vi "CoordToMeters.vi"(10 "Ref Point":cluster{"Lat":dbl, "Long":dbl} {"Long" format="%#.22g"; "Lat" format="%#.22g"}, 11 "GPS position":cluster{"Lat":dbl, "Long":dbl} {"Long" format="%#.22g"; "Lat" format="%#.22g"}) -> (2 "X":dbl format="%#.14g", 3 "Y":dbl format="%#.14g")   [LabVIEW 2016]
uses:
  <vilib>/imath/engines/lvmath2/RunTimeEngine/NodeEndStatement/NIMS_NodeEndStatement_Output.vi
  <instcachedir>/0/NIMS_NodeEndStatement_Output_53EC0D466D134D7ABD903AC30B43404B.lvgen/NIMS_NodeEndStatement_Output_53EC0D466D134D7ABD903AC30B43404B_001.vi
  <vilib>/imath/engines/lvmath2/RunTimeEngine/ErrorHandling/NIMS_Finalize Error.vi
panel:
  out "Distance to the reference point":dbl format="%#.22g"
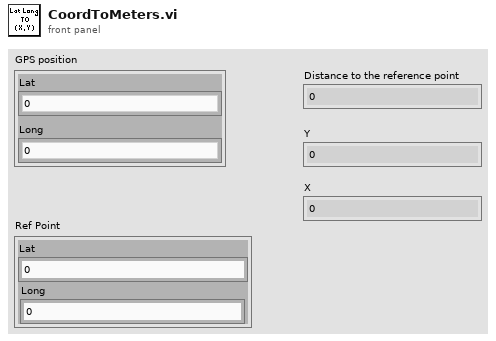
[diagram p1: front panel]
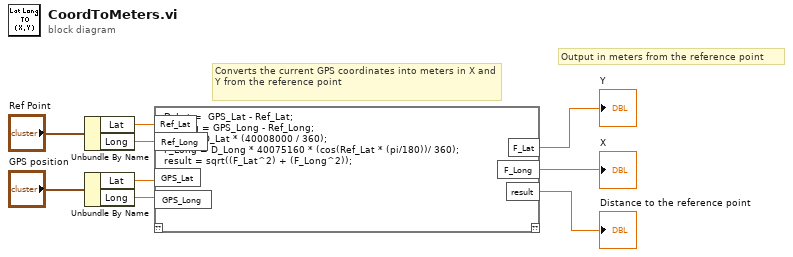
[diagram p0: block diagram]
diagram:
  # "Output in meters from the reference point"
  # "Converts the current GPS coordinates into meters in X and Y from the reference point"
  n1 = Unbundle By Name("Ref Point") -> ("Lat"=w6:dbl, "Long"=w5:dbl)
  n2 = Unbundle By Name("GPS position") -> ("Lat"=w2:dbl, "Long"=w1:dbl)
  n3 = mathscript code="D_Lat =  GPS_Lat - Ref_Lat;\nD_Long = GPS_Long - Ref_Long;\nF_Lat = D_Lat * (40008000 / 360);\nF_Long = D_Long * 40075160 * (cos(Ref_Lat * (pi/180))/ 360);\nresult = sqrt((F_Lat^2) + (F_Long^2));"("Ref_Lat"=w6, "Ref_Long"=w5, "GPS_Lat"=w2, "GPS_Long"=w1) -> ("result"=→"Distance to the reference point":dbl, "F_Lat"=→"Y":dbl, "F_Long"=→"X":dbl)  [unwired: 1 in, 1 out]
